vi "AAA Device Level, Catalog.vi"   [LabVIEW 2010]
uses:
  Active Output Test Cases.ctl
  Generic/Waveform Attribute/Waveform Attribute Cluster.ctl
  Analyze Ouptut Parameters.ctl
panel:
  # "Device Level\nCatalog"
types:
  T1 = typedef "Analyze Ouptut Parameters.ctl" = cluster{"Stim Amplitude":dbl[], "Stim Pulse Width":dbl[], "Interphase Delay":dbl[], "Recovery Amplitude":dbl[], "Recovery PW":dbl[], "Recovery Holdoff":dbl[], "Frequency":dbl, "Avg CBC Width":dbl, "Avg. CBC Holdoff":dbl, "Avg. CBC Amplitude":dbl}
  T2 = cluster{"Pulses per Cycle":i32, "Load Resistance (Ohms)":dbl, "Krec Value":i32, "Recovery Mode (T=Active)":bool, "Target Stim Currents (Amps)":dbl[]}
  T3 = typedef "Waveform Attribute Cluster.ctl" = cluster{"Label":string, "Value":dbl}
  T4 = typedef "Active Output Test Cases.ctl" = enum16{"TC1", "TC2", "TC3", "TC4", "TC5", "TC6", "TC7", "TC8", "TC9", "TC10", "TC11", "TC12", "TC13", "TC14", "TC15", "TC16", "TC17", "TC18", "TC19", "TC20", "TC21", "TC22", "TC23", "TC24", "TC25", "TC26", "TC27", "TC28", "TC29", "TC30", "TC31", "TC32", "TC33", "TC34", "TC35", "TC36"}
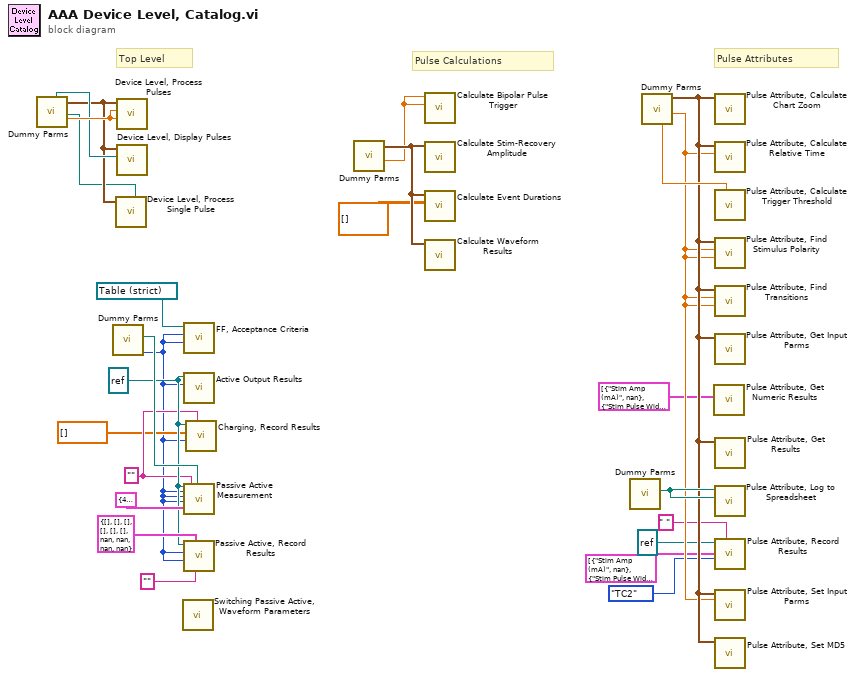
[diagram p0: block diagram]
diagram:
  w3 = "" ("step name")
  w4 = refnum<k7> refnum ("Sequence Context")
  # "Pulse Attributes"
  # "Pulse Calculations"
  # "Top Level"
  n1 = call "Dummy Parms.vi"() -> ("DBL"=w25:dbl, "path"=w15:path, "waveform"=w16:waveform(dbl), "WFG Refnum"=w24:refnum<vi>)  [unwired: 6 in, 2 out]
  n2 = call "Dummy Parms.vi"() -> ("I32"=w1:i32, "path"=w8:path)  [unwired: 6 in, 4 out]
  n3 = call "Device Level, Process Single Pulse.vi"("filepath"=w15, "waveform array"=w16) -> ()  [unwired: 6 in, 4 out]
  n4 = call "Device Level, Process Pulses.vi"("Average Size"=w25, "Resistance (ohms)"=w25, "waveform"=w16) -> ()  [unwired: 3 in, 4 out]
  n5 = call "Device Level, Display Pulses.vi"("WFGraph Refnum"=w24, "waveform"=w16) -> ()  [unwired: 7 in, 2 out]
  n6 = call "Switching Passive Active, Waveform Parameters.vi"() -> ()  [unwired: 9 in, 2 out]
  n7 = call "FF, Acceptance Criteria.vi"("n rows"=w1, "test case"=w1, "Tbl Refnum"=refnum<vi> refnum) -> ()  [unwired: 7 in, 2 out]
  n8 = call "Active Output Results.vi"("test case"=w1, "Sequence Context"=w4) -> ()  [unwired: 8 in, 2 out]
  n9 = call "Passive Active Measurement.vi"("Sequence Context"=w4, "test case"=w1, "n rows"=w1, "Idle Offset Voltage"=w1, "Pulse Characteristics"=T2 {"Pulses per Cycle"=4, "Load Resistance (Ohms)"=nan, "Krec Value"=2, "Recovery Mode (T=Active)"=TRUE, "Target Stim Currents (Amps)"=[]}, "step name"=w3, "filepath"=w8) -> ()  [unwired: 12 in, 1 out]
  n10 = call "Passive Active, Record Results.vi"("step name"="", "Waveform Parameters"=T1 {"Stim Amplitude"=[], "Stim Pulse Width"=[], "Interphase Delay"=[], "Recovery Amplitude"=[], "Recovery PW"=[], "Recovery Holdoff"=[], "Frequency"=nan, "Avg CBC Width"=nan, "Avg. CBC Holdoff"=nan, "Avg. CBC Amplitude"=nan}, "n rows"=w1, "test case"=w1, "Sequence Context"=w4) -> ()  [unwired: 5 in, 2 out]
  n11 = call "Charging, Record Results.vi"("step name"=w3, "test case"=w1, "Numeric Results"=dbl[] [] ("transitions"), "Sequence Context"=w4) -> ()  [unwired: 6 in, 2 out]
  n12 = call "Dummy Parms.vi"() -> ("DBL"=w18:dbl, "waveform"=w19:waveform(dbl))  [unwired: 6 in, 4 out]
  n13 = call "Calculate Bipolar Pulse Trigger.vi"("Recvy Amp (V)"=w18, "Stim Amp (V)"=w18) -> ()  [unwired: 6 in, 4 out]
  n14 = call "Calculate Stim-Recovery Amplitude.vi"("waveform"=w19) -> ()  [unwired: 7 in, 4 out]
  n15 = call "Calculate Event Durations.vi"("transitions"=dbl[][] [], "waveform"=w19) -> ()  [unwired: 8 in, 2 out]
  n16 = call "Calculate Waveform Results.vi"("waveform in"=w19) -> ()  [unwired: 9 in, 2 out]
  n17 = call "Dummy Parms.vi"() -> ("path"=w23:path)  [unwired: 6 in, 5 out]
  n18 = call "Dummy Parms.vi"() -> ("DBL"=w20:dbl, "waveform"=w21:waveform(dbl), "DBL volts"=w22:dbl[unit])  [unwired: 6 in, 3 out]
  n19 = call "Pulse Attribute, Get Numeric Results.vi"("results"=T3[] [{"Label"="Stim Amp (mA)", "Value"=nan}, {"Label"="Stim Pulse Width (us)", "Value"=nan}, {"Label"="Interphase Delay (us)", "Value"=nan}, {"Label"="Recvy Amp (mA)", "Value"=nan}, {"Label"="Recvy Pulse Width (us)", "Value"=nan}, {"Label"="Frequency (Hz)", "Value"=nan}, {"Label"="Period Jitter (us rms)", "Value"=nan}]) -> ()  [unwired: 5 in, 2 out]
  n20 = call "Pulse Attribute, Calculate Chart Zoom.vi"("waveform"=w21) -> ()  [unwired: 3 in, 8 out]
  n21 = call "Pulse Attribute, Calculate Relative Time.vi"("index"=w20, "waveform"=w21) -> ()  [unwired: 5 in, 3 out]
  n22 = call "Pulse Attribute, Calculate Trigger Threshold.vi"("pulse amp"=w22) -> ()  [unwired: 6 in, 2 out]
  n23 = call "Pulse Attribute, Find Stimulus Polarity.vi"("amp min"=w20, "amp max"=w20, "waveform"=w21) -> ()  [unwired: 5 in, 4 out]
  n24 = call "Pulse Attribute, Find Transitions.vi"("Recvy Amp (V)"=w20, "Stim Amp (V)"=w20, "waveform"=w21) -> ()  [unwired: 6 in, 3 out]
  n25 = call "Pulse Attribute, Get Input Parms.vi"("waveform"=w21) -> ()  [unwired: 6 in, 3 out]
  n26 = call "Pulse Attribute, Get Results.vi"("waveform"=w21) -> ()  [unwired: 6 in, 3 out]
  n27 = call "Pulse Attribute, Log to Spreadsheet.vi"("results file"=w23, "waveform file"=w23) -> ()  [unwired: 7 in, 1 out]
  n28 = call "Pulse Attribute, Record Results.vi"("step name"=" ", "test case"=Active_Output_Test_Cases."TC2", "results"=T3[] [{"Label"="Stim Amp (mA)", "Value"=nan}, {"Label"="Stim Pulse Width (us)", "Value"=nan}, {"Label"="Interphase Delay (us)", "Value"=nan}, {"Label"="Recvy Amp (mA)", "Value"=nan}, {"Label"="Recvy Pulse Width (us)", "Value"=nan}, {"Label"="Frequency (Hz)", "Value"=nan}, {"Label"="Period Jitter (us rms)", "Value"=nan}], "Sequence Context"=refnum<k7> refnum) -> ()  [unwired: 6 in, 2 out]
  n29 = call "Pulse Attribute, Set Input Parms.vi"("Average Size"=w20, "Resistance (ohms)"=w20, "waveform"=w21) -> ()  [unwired: 5 in, 2 out]
  n30 = call "Pulse Attribute, Set MD5.vi"("waveform"=w21) -> ()  [unwired: 4 in, 5 out]
